vi "Teardown.vi"(11 "Base Event Actor in":refnum<class "Base Event Actor.lvclass">) -> (3 "Base Event Actor out":refnum<class "Base Event Actor.lvclass">)   [LabVIEW 2021, in "jettl.lvlib" / "Base Event Actor.lvclass"]
uses:
  Base Event Actor.lvclass
  Event State/Teardown Event State/Teardown Event State.lvclass
  C:/git/jettl/src/jettl/Event State/Event State/Event State.lvclass
  Base Event Actor.lvclass/Base Event Actor.ctl
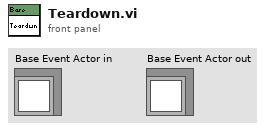
[diagram p1: front panel]
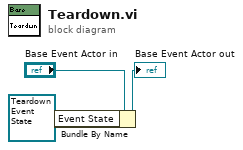
[diagram p0: block diagram]
diagram:
  n1 = Bundle By Name(cluster="Base Event Actor in", "Event State"=refnum<class "Teardown Event State.lvclass"> refnum ("jettl.lvlib:Teardown Event State.lvclass")) -> (→"Base Event Actor out":refnum<class "Base Event Actor.lvclass">)
